vi "Get value.vi"(11 "ExpFitter in":refnum<class "ExpFitter.lvclass">) -> (0 "residue":dbl, 1 "offset":dbl, 2 "damping":dbl, 3 "amplitude":dbl)   [LabVIEW 2019, in "ExpFitter.lvclass"]
uses:
  ExpFitter.lvclass
  ExpFitter.lvclass/ExpFitter.ctl
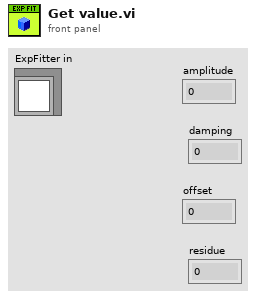
[diagram p1: front panel]
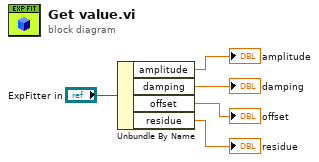
[diagram p0: block diagram]
diagram:
  n1 = Unbundle By Name("ExpFitter in") -> ("amplitude"=→"amplitude":dbl, "damping"=→"damping":dbl, "offset"=→"offset":dbl, "residue"=→"residue":dbl)
